vi "Remove Connection.vi"(8 "error in (no error)":errorcluster, 10 "ID":i32, 11 "Connection Listener in":refnum<class "Connection Listener.lvclass">) -> (0 "error out":errorcluster, 3 "Connection Listener out":refnum<class "Connection Listener.lvclass">)   [LabVIEW 2017, in "Connection Listener.lvlib" / "Connection Listener.lvclass"]
uses:
  Connection Listener.lvclass
  Connection Listener.lvclass/Connection Listener.ctl
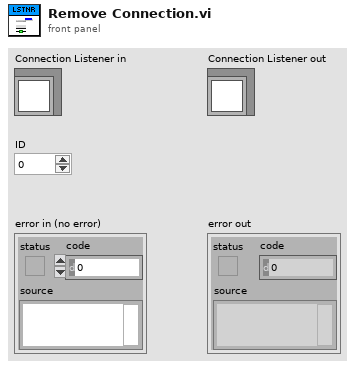
[diagram p1: front panel]
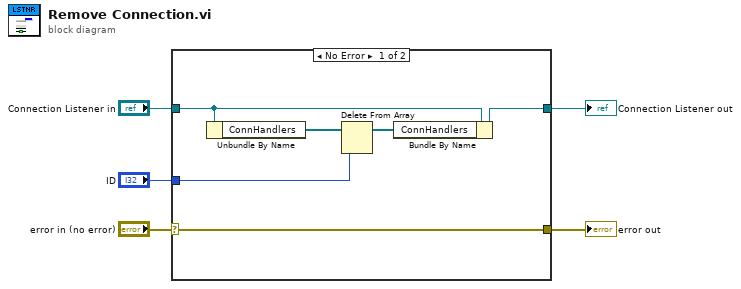
[diagram p0: block diagram]
diagram:
  n1 = case shown="No Error" "error in (no error)" {
    selector: "error in (no error)" -> [w6 w13]
    tunnel: [w6 w13] -> w4
    tunnel: [w11 w12] -> w2
    tunnel: "Connection Listener in" -> [w8 w12]
    tunnel: "ID" -> [w7 _]
    frame No Error {
      n2 = Unbundle By Name(w8) -> ("ConnHandlers"=w10:refnum<class "Message Enqueuer.lvclass">[])
      n3 = Delete From Array(array=w10, index=w7) -> (array with subset deleted=w9:refnum<class "Message Enqueuer.lvclass">[])  [unwired: 1 in, 1 out]
      n4 = Bundle By Name(cluster=w8, "ConnHandlers"=w9) -> (w11:refnum<class "Connection Listener.lvclass">)
    }
    frame Error {
    }
  }
  "error out" <- w4
  "Connection Listener out" <- w2
